vi "populateILCMap.vi"(8 "error in (no error)":errorcluster, 11 "ILCCommunications in":refnum<class "ILCCommunications.lvclass">) -> (0 "error out":errorcluster, 3 "ILCCommunications out":refnum<class "ILCCommunications.lvclass">)   [LabVIEW 2016, in "ILCCommunications.lvclass"]
uses:
  ILCCommunications.lvclass
  Types/ILCMap.ctl
  Types/ILCTypes.ctl
  ILCCommunications.lvclass/ILCCommunications.ctl
  Types/M1M3SupportTypes.lvlib
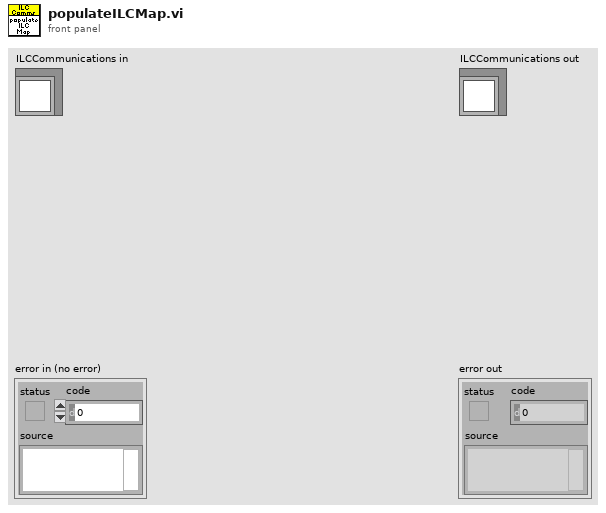
[diagram p1: front panel]
types:
  T1 = typedef "M1M3SupportTypes.lvlib/ILCMap.ctl" = cluster{"Index":i32, "Type":T2}
  T2 = typedef "M1M3SupportTypes.lvlib/ILCTypes.ctl" = enum16{"Hardpoint", "Force"}
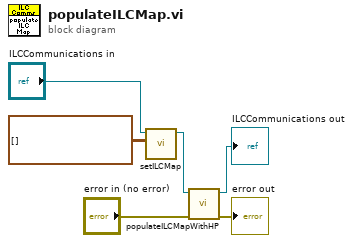
[diagram p0: block diagram]
diagram:
  n1 = call "setILCMap.vi"("ILCMap"=T1[][] [], "ILCCommunications in"="ILCCommunications in") -> ("ILCCommunications out"=w4:refnum<class "ILCCommunications.lvclass">)  [unwired: 9 in]
  n2 = call "populateILCMapWithHP.vi"("error in (no error)"="error in (no error)", "ILCCommunications in"=w4) -> ("error out"=→"error out":errorcluster, "ILCCommunications out"=→"ILCCommunications out":refnum<class "ILCCommunications.lvclass">)  [unwired: 8 in]
